vi "Demo HAL Tester LITE.vi"() -> ()   [LabVIEW 2014]
doc: "Use this template to build a producer/consumer design pattern with events to produce queue items. Use this design pattern instead of the User Interface Event Handler pattern for user interfaces when you want to execute code asynchronously in response to an event without slowing the user interface responsiveness."
uses:
  TypeDefs/HAL Config Data.ctl
  APIs/Message Queue/Enqueue Message (Single).vi
  APIs/Message Queue/Enqueue Message (Array).vi
  APIs/Message Queue/WINFAS 2 Message Queue.lvlib
  HWSyncLoop/HWSyncLoop.lvlib
  APIs/Data Queue/WINFAS 2 Data Queue.lvlib
  HWAsyncLoop/HWAsyncLoop.lvlib
panel:
  out "Asyncs":string[][](array[string])
  out "Syncs":string[](array[string])
  out "Async Data":sgl[](array[numeric])
  in  "HWAsync CMD":bool
  in  "HWSync CMD":bool
  in  "Stop Cycle":bool
  in  "Start Cycle":bool
  in  "Config":bool
  in  "LOAD DRIVER":bool
  in  "Disconnect":bool
  in  "Connect":bool
  out "UI Mssge Log":string
  out "TDX":sgl[][](graph)
  out "Encoder":sgl[](array[slide]) scale=-3600.0..3600.0
  out "DO":bool[][](array[boolean])
  out "DI":bool[][](array[boolean])
  out "TDX ALL":string[][](table)
  out "HWSyncLog 1":string
  out "HWSyncLog 2":string
  out "HWSyncLog 3":string
  out "HWSyncLog 4":string
  out "HWSyncLog 5":string
  out "HWAsyncLogAll":string
  # "Entradas Digitales (0-15)"
  # "Salidas Digitales (0-15)"
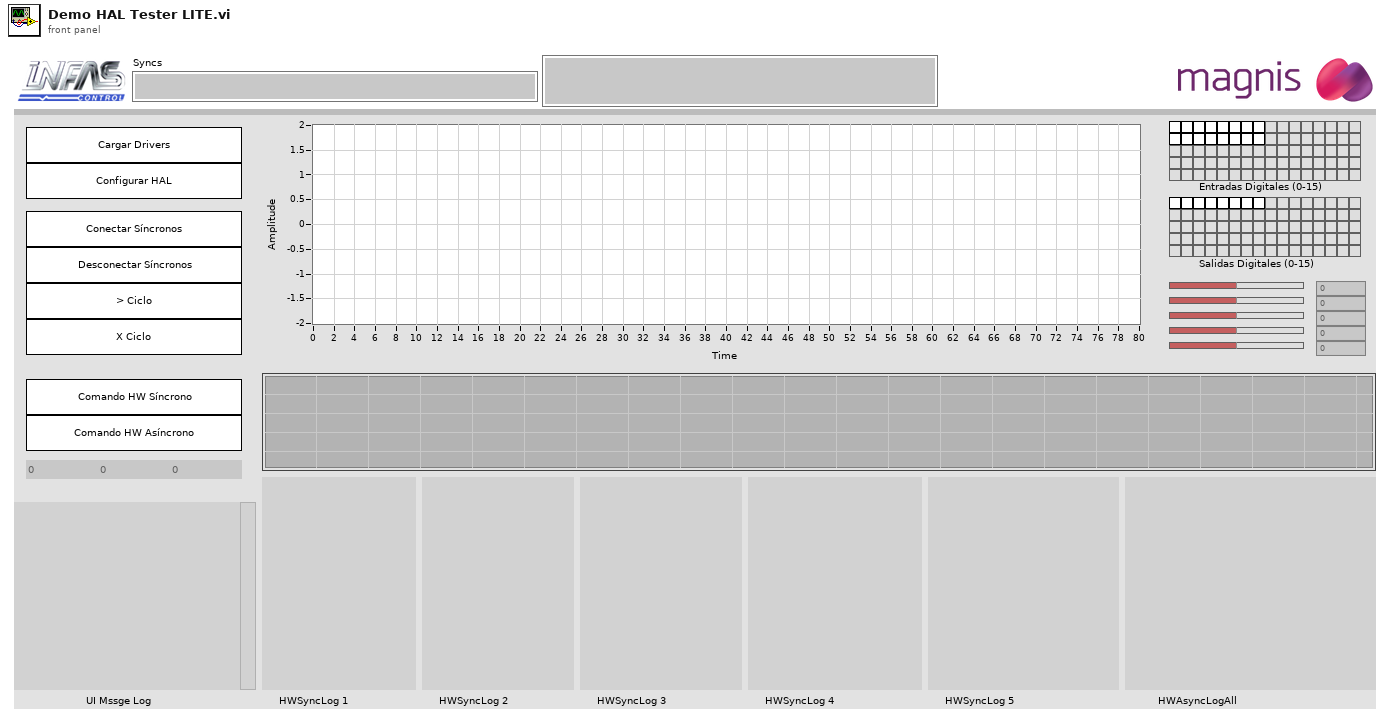
[diagram p1: front panel]
types:
  T1 = typedef "HAL Config Data.ctl" = cluster{"HWSync Index":u32, "Driver Name":string, "Channel Mask":u64}
  T2 = enum32{"invalid app kind", "Development System", "Run Time System", "Student Edition", "Embedded LabVIEW", "Evaluation", "Custom"}
  T3 = typedef "WINFAS 2 Message Queue.lvlib/All Message Queues.ctl" = cluster{"CORE":refnum<queue>, "Event UI":refnum<queue>, "Display UI":refnum<queue>, "MATH":refnum<queue>, "SEQ":refnum<queue>, "DB":refnum<queue>, "ERR":refnum<queue>, "HAL":refnum<queue>, "HWSync1":refnum<queue>, "HWSync2":refnum<queue>, "HWSync3":refnum<queue>, "HWSync4":refnum<queue>, "HWSync5":refnum<queue>, "HWAsync1":refnum<queue>, "HWAsync2":refnum<queue>, "HWAsync3":refnum<queue>, "HWAsync4":refnum<queue>, "HWAsync5":refnum<queue>, "HWAsync6":refnum<queue>, "HWAsync7":refnum<queue>, "HWAsync8":refnum<queue>, "HWAsync9":refnum<queue>, "HWAsync10":refnum<queue>}
  T4 = typedef "WINFAS 2 Data Queue.lvlib/All Data Queues Cluster.ctl" = cluster{"Queues":cluster{"ACQ HWSync1":refnum<queue>, "ACQ HWSync2":refnum<queue>, "ACQ HWSync3":refnum<queue>, "ACQ HWSync4":refnum<queue>, "ACQ HWSync5":refnum<queue>}, "Notifiers":cluster{"Control":cluster{"CTRL HWSync1":refnum<notifier>, "CTRL HWSync2":refnum<notifier>, "CTRL HWSync3":refnum<notifier>, "CTRL HWSync4":refnum<notifier>, "CTRL HWSync5":refnum<notifier>}, "Acquisition":cluster{"ACQ HWSync1":refnum<notifier>, "ACQ HWSync2":refnum<notifier>, "ACQ HWSync3":refnum<notifier>, "ACQ HWSync4":refnum<notifier>, "ACQ HWSync5":refnum<notifier>}, "Async":cluster{"ACQ HWAsync1":refnum<notifier>, "ACQ HWAsync2":refnum<notifier>, "ACQ HWAsync3":refnum<notifier>, "ACQ HWAsync4":refnum<notifier>, "ACQ HWAsync5":refnum<notifier>, "ACQ HWAsync6":refnum<notifier>, "ACQ HWAsync7":refnum<notifier>, "ACQ HWAsync8":refnum<notifier>, "ACQ HWAsync9":refnum<notifier>, "ACQ HWAsync10":refnum<notifier>}}}
  T5 = cluster{"ACQ HWSync1":refnum<notifier>, "ACQ HWSync2":refnum<notifier>, "ACQ HWSync3":refnum<notifier>, "ACQ HWSync4":refnum<notifier>, "ACQ HWSync5":refnum<notifier>}
  T6 = cluster{"CTRL HWSync1":refnum<notifier>, "CTRL HWSync2":refnum<notifier>, "CTRL HWSync3":refnum<notifier>, "CTRL HWSync4":refnum<notifier>, "CTRL HWSync5":refnum<notifier>}
  T7 = cluster{"ACQ HWSync1":refnum<queue>, "ACQ HWSync2":refnum<queue>, "ACQ HWSync3":refnum<queue>, "ACQ HWSync4":refnum<queue>, "ACQ HWSync5":refnum<queue>}
  T8 = cluster{"HWSync1":refnum<queue>, "HWSync2":refnum<queue>, "HWSync3":refnum<queue>, "HWSync4":refnum<queue>, "HWSync5":refnum<queue>}
  T9 = cluster{"HWAsync1":refnum<queue>, "HWAsync2":refnum<queue>, "HWAsync3":refnum<queue>, "HWAsync4":refnum<queue>, "HWAsync5":refnum<queue>, "HWAsync6":refnum<queue>, "HWAsync7":refnum<queue>, "HWAsync8":refnum<queue>, "HWAsync9":refnum<queue>, "HWAsync10":refnum<queue>}
  T10 = typedef "WINFAS 2 Data Queue.lvlib/Async Acquisition Data Cluster.ctl" = cluster{"Data":sgl[]}
  T11 = typedef "WINFAS 2 Data Queue.lvlib/Acquisition Data 1 Sample Cluster.ctl" = cluster{"TDX":sgl[], "Encoder":sgl}
  T12 = typedef "WINFAS 2 Data Queue.lvlib/Control Data Cluster.ctl" = cluster{"Encoder":sgl, "DI":bool[], "DO":bool[]}
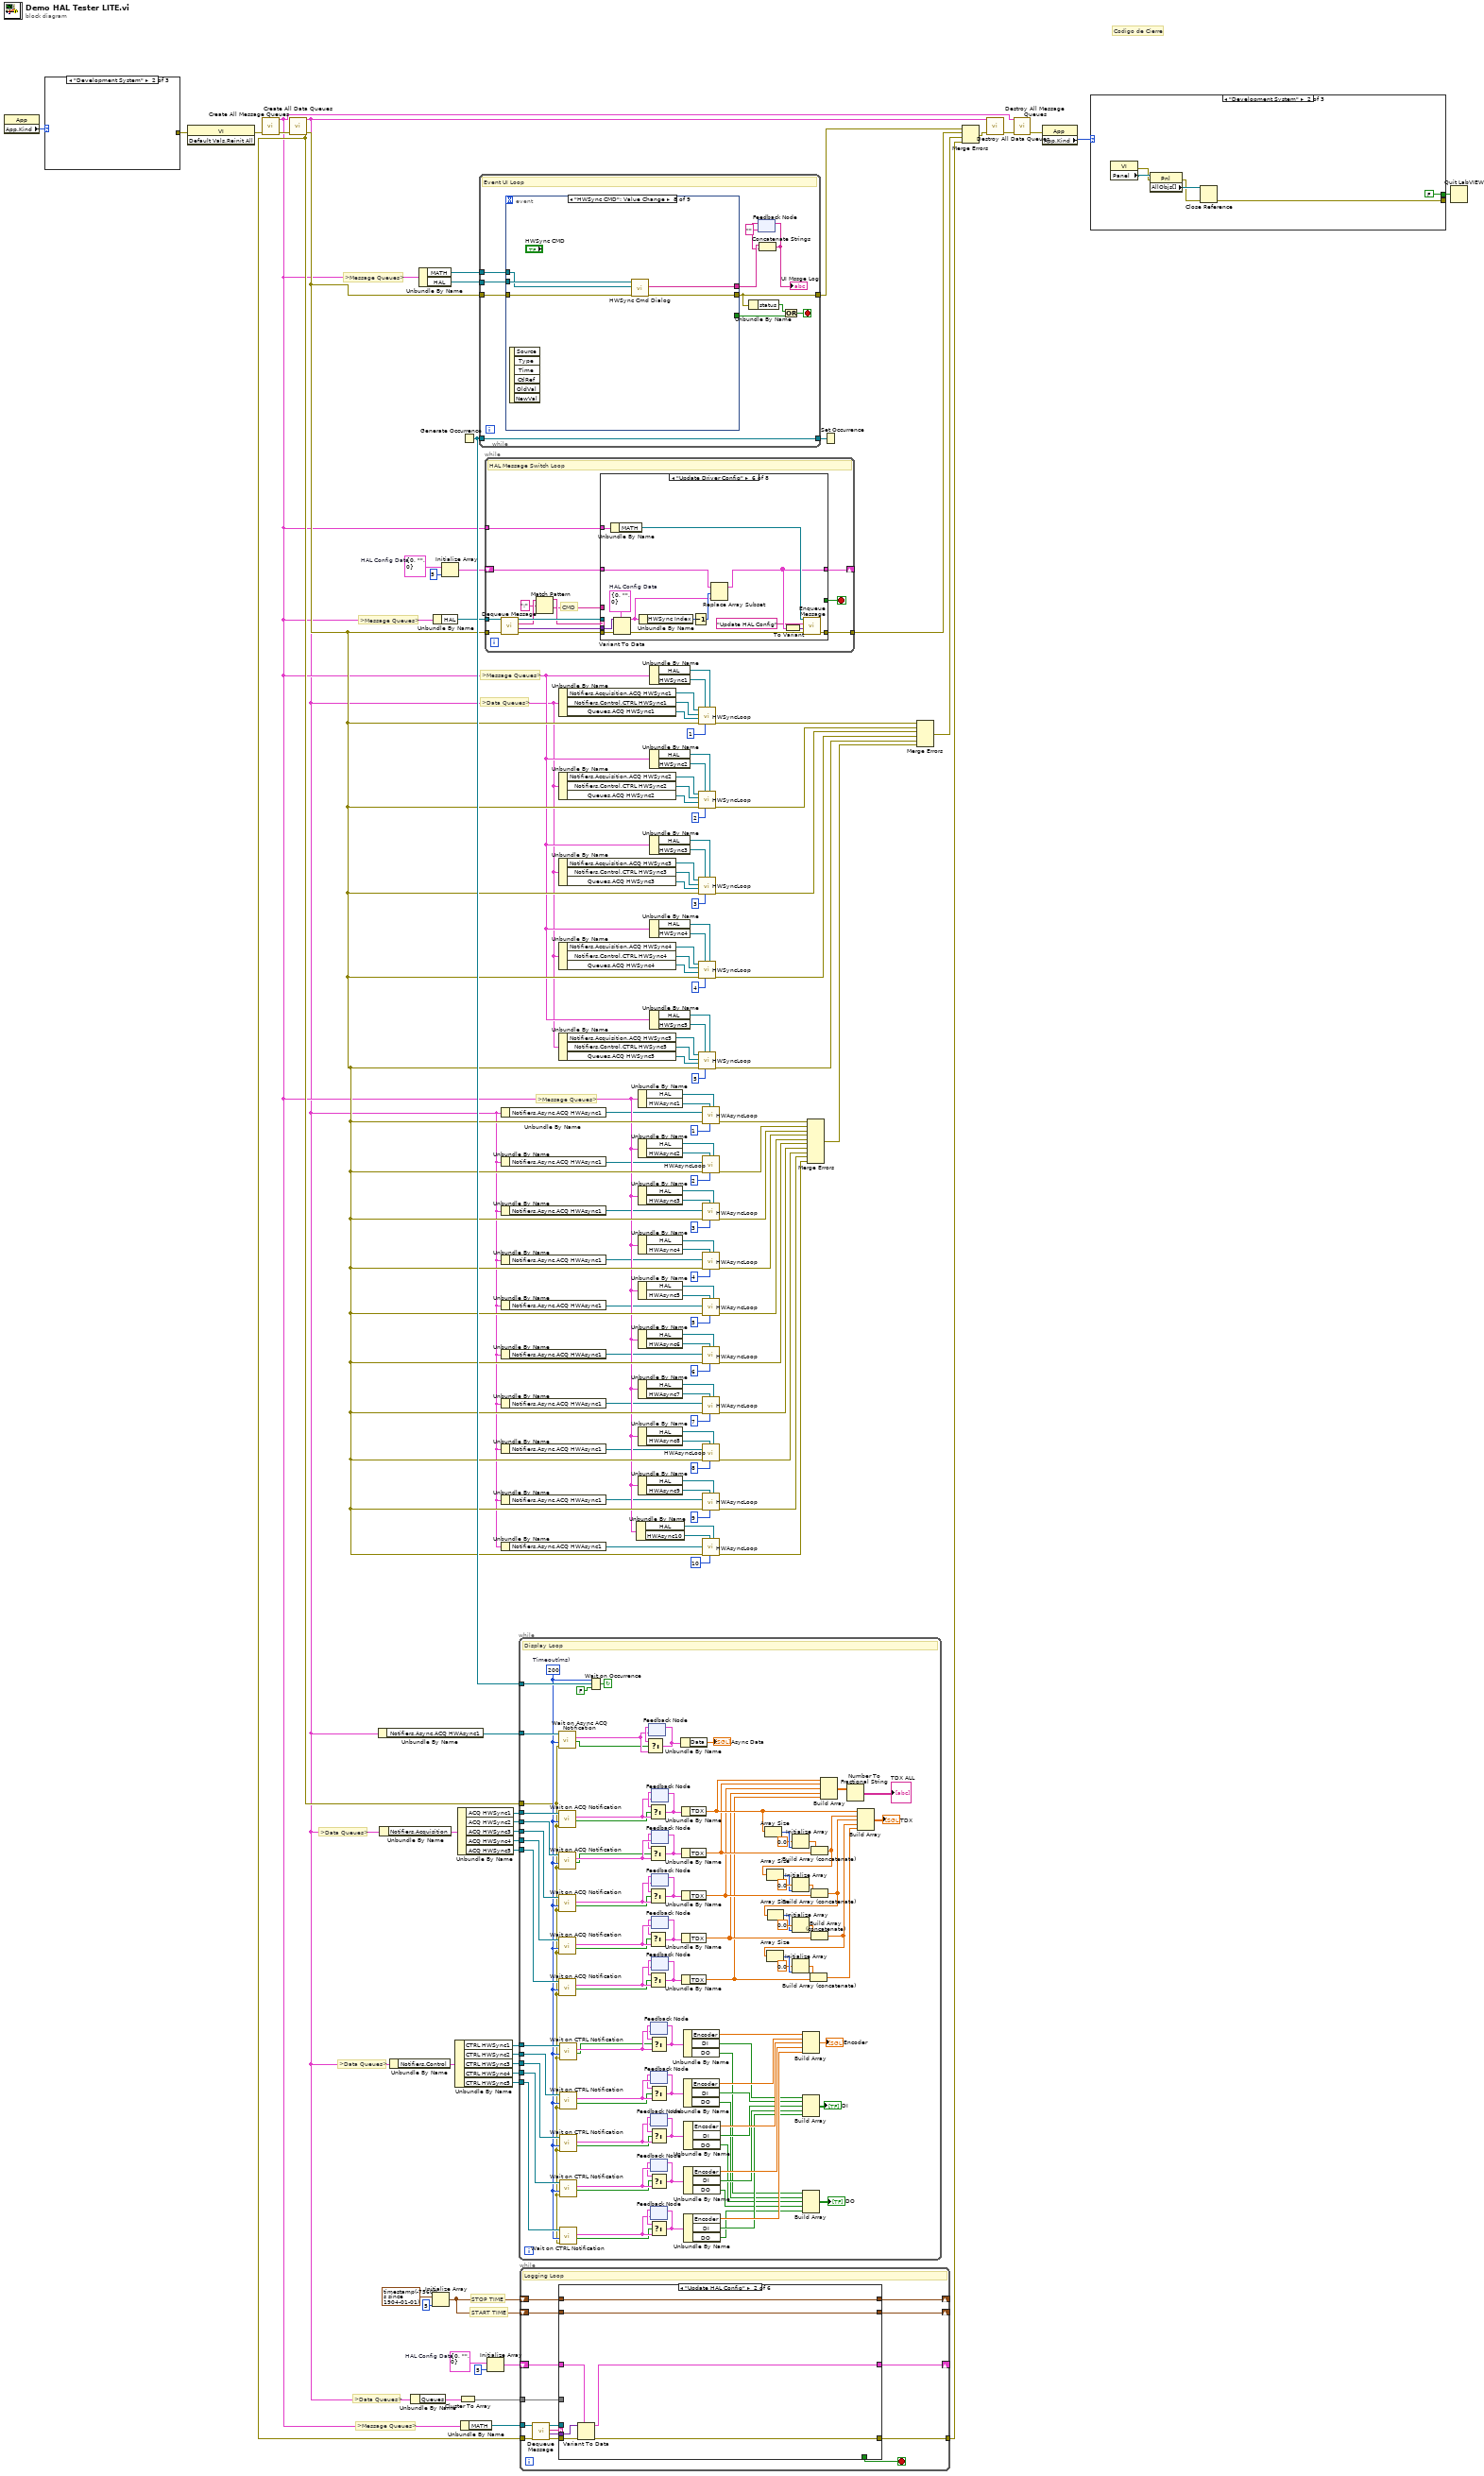
[diagram p0: block diagram]
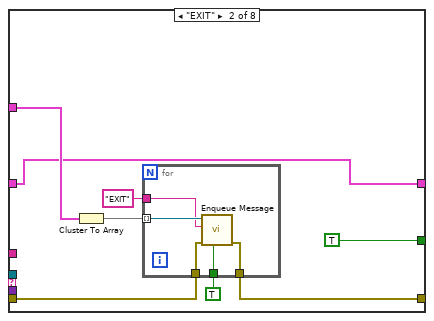
[diagram p3: hidden frame]
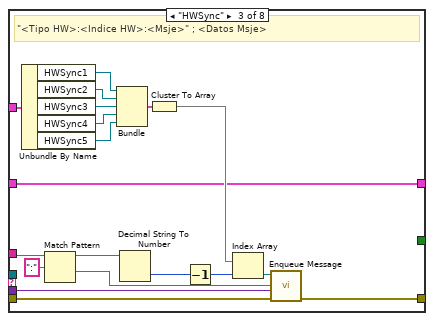
[diagram p4: hidden frame]
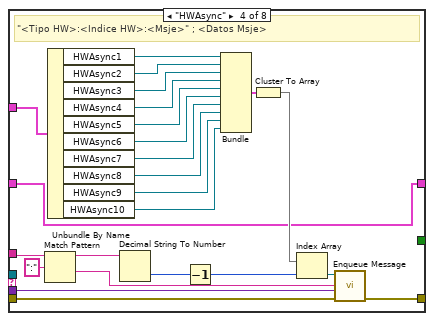
[diagram p5: hidden frame]
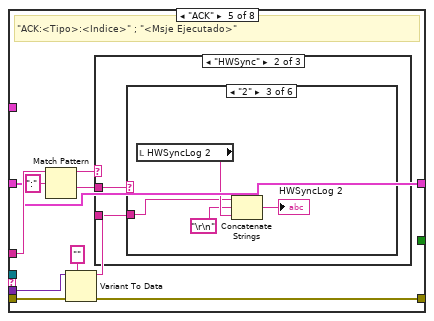
[diagram p6: hidden frame]
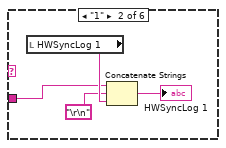
[diagram p9: hidden frame]
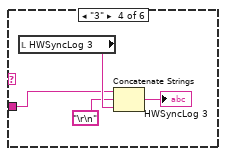
[diagram p10: hidden frame]
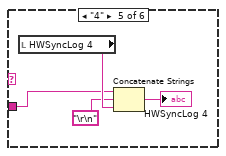
[diagram p11: hidden frame]
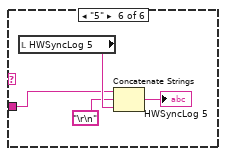
[diagram p12: hidden frame]
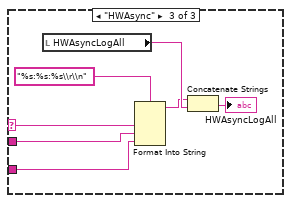
[diagram p13: hidden frame]
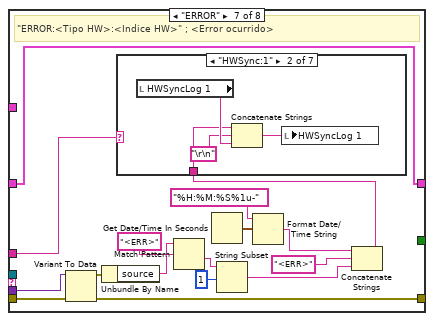
[diagram p14: hidden frame]
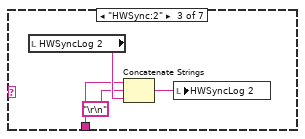
[diagram p16: hidden frame]
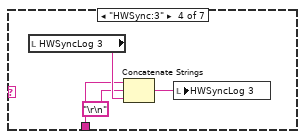
[diagram p17: hidden frame]
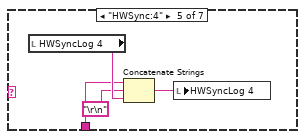
[diagram p18: hidden frame]
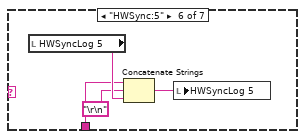
[diagram p19: hidden frame]
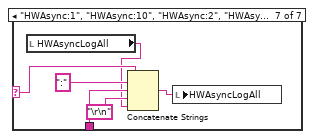
[diagram p20: hidden frame]
diagram:
  w17 = T1 {"HWSync Index"=0, "Driver Name"="", "Channel Mask"=0}  # HAL Config Data
  w20 = T1 {"HWSync Index"=0, "Driver Name"="", "Channel Mask"=0}  # HAL Config Data
  # "START TIME"
  # "STOP TIME"
  # ">Message Queues>"
  # ">Message Queues>"
  # ">Data Queues>"
  # "Codigo de Cierre"
  # ">Message Queues>"
  # ">Data Queues>"
  # ">Message Queues>"
  # ">Data Queues>"
  # ">Data Queues>"
  # ">Message Queues>"
  n1 = property class="App"() -> ("App.Kind"=w123:T2)  [unwired: 2 in, 2 out]
  n2 = case shown="\"Development System\"" w123 {
    tunnel: [_ _ w134] -> w122
    frame "invalid app kind", Default {
    }
    frame "Development System" {
    }
    frame "Run Time System" {
      w133 = FALSE ("Front Panel Window:Show Menu Bar")
      n3 = invoke class="VI" method="FP.Run-Time Position.Maximized"("Monitor"=i16 0) -> (error out=w134:errorcluster)  [unwired: 3 in, 3 out]
      n4 = property class="VI"("Front Panel.ShowMenuBar"=w133, "TB.Visible"=w133) -> ()  [unwired: 2 in, 2 out]
    }
  }
  n5 = invoke class="VI" method="Default Vals.Reinit All"(error in=w122) -> (error out=w113:errorcluster)  [unwired: 2 in, 2 out]
  n6 = call "Create All Message Queues.vi"("error in (no error)"=w113) -> ("error out"=w114:errorcluster, "Message Queues Out"=w24:T3)  [unwired: 9 in]
  n7 = call "Create All Data Queues.vi"("Error In"=w114) -> ("Error Out"=w36:errorcluster, "WINFAS 2 Data Queue.lvlib:All Data Queues Cluster"=w2:T4)  [unwired: 9 in]
  n8 = Unbundle By Name(w2) -> ("Notifiers.Async.ACQ HWAsync1"=w1:refnum<notifier>)
  n9 = Unbundle By Name(w2) -> ("Notifiers.Acquisition"=w68:T5)
  n10 = Unbundle By Name(w2) -> ("Notifiers.Control"=w67:T6)
  n11 = Unbundle By Name(w2) -> ("Queues"=w14:T7)
  n12 = Unbundle By Name(w24) -> ("MATH"=w132:refnum<queue>, "HAL"=w128:refnum<queue>)
  n13 = Initialize Array(timestamp(-75600 s since 1904-01-01) ("current time"), 5 ("dimension size")) -> (w21:timestamp[])
  n14 = Unbundle By Name(w24) -> ("HAL"=w72:refnum<queue>)
  n15 = Initialize Array(w17, 5 ("dimension size")) -> (w15:T1[])
  n16 = Unbundle By Name(w67) -> ("CTRL HWSync1"=w77:refnum<notifier>, "CTRL HWSync2"=w76:refnum<notifier>, "CTRL HWSync3"=w75:refnum<notifier>, "CTRL HWSync4"=w74:refnum<notifier>, "CTRL HWSync5"=w73:refnum<notifier>)
  n17 = Unbundle By Name(w68) -> ("ACQ HWSync1"=w118:refnum<notifier>, "ACQ HWSync2"=w81:refnum<notifier>, "ACQ HWSync3"=w80:refnum<notifier>, "ACQ HWSync4"=w79:refnum<notifier>, "ACQ HWSync5"=w78:refnum<notifier>)
  n18 = Cluster To Array(cluster=w14) -> (array=w13:refnum<queue>[])
  n19 = Unbundle By Name(w24) -> ("MATH"=w126:refnum<queue>)
  n20 = Generate Occurrence() -> (w111:refnum<k4>)
  n21 = while {
    tunnel: w132 -> [w147]
    tunnel: w128 -> [w142]
    tunnel: [w140] -> w112
    tunnel: w111 -> [w140]
    tunnel: w36 -> [w146]
    tunnel: [w144] -> w129
    stop <- w141 stop-if-true
    # "Event UI Loop"
    n22 = event shown="[7] \"HWSync CMD\": Value Change" {
      selector: _ -> [_ _ _ _ _ _ _ _ _]
      dyn-events: _ -> [_ _ _ _ _ _ _ _ _]
      timeout: _ -> [_ _ _ _ _ _ _ _ _]
      tunnel: w147 -> [w153 _ _ _ _ _ w212 w227 _]
      tunnel: w146 -> [w155 w165 w171 w180 w187 w194 w211 w231 w237]
      tunnel: [w150 w163 w170 w179 w186 w192 w216 w230 w235] -> w144
      tunnel: [TRUE ("stop") _ _ _ _ _ _ _ _] -> w145
      tunnel: w142 -> [w156 w164 w169 w178 w185 w193 w217 w229 w232]
      tunnel: [_ w162 w166 w175 w184 w189 w215 w228 w234] -> w139
      event Panel Close? {
        w154 = TRUE ("Priority Message? (F)")
        w152 = "EXIT" ("String")
        n23 = event-data() -> ()  [unwired: 1 in, 1 out]
        n24 = call-poly "Enqueue Message.vi"("Priority Message? (F)"=w154, "error in (no error)"=w155, "Message"=w152, "Message Queue"=w156) -> ("error out"=w151:errorcluster)  [unwired: 6 in, 1 out]
        n25 = call-poly "Enqueue Message.vi"("Priority Message? (F)"=w154, "error in (no error)"=w151, "Message"=w152, "Message Queue"=w153) -> ("error out"=w150:errorcluster)  [unwired: 6 in, 1 out]
        n26 = event-data("Discard?"=TRUE) -> ()  [unwired: 1 in, 1 out]
      }
      event "LOAD DRIVER": Value Change {
        n27 = event-data() -> ()  [unwired: 1 in, 1 out]
        n28 = call "Load Drivers Dialog.vi"("error in (no error)"=w165, "Message Queue in"=w164) -> ("error out"=w163:errorcluster, "Mssgs Sent"=w162:string, "Asyncs"=w160:string[], "Syncs"=→"Syncs":string[])  [unwired: 6 in]
        n29 = Reshape Array(w160, 2 ("dimension size"), 5 ("dimension size")) -> (→"Asyncs":string[][])
      }
      event "Connect": Value Change {
        w168 = string[] ["HWSync:1:Port:Open", "HWSync:2:Port:Open", "HWSync:3:Port:Open", "HWSync:4:Port:Open", "HWSync:5:Port:Open"] ("Message Array")
        n30 = event-data() -> ()  [unwired: 1 in, 1 out]
        n31 = for {
          tunnel: [w174] -> w167 mode=indexing
          tunnel: w168 -> [w173] mode=indexing
          n32 = Concatenate Strings(w173, "\r\n") -> (w174:string)
        }
        n33 = call-poly "Enqueue Message.vi"("error in (no error)"=w171, "Message Array"=w168, "Message Queue"=w169) -> ("error out"=w170:errorcluster)  [unwired: 7 in, 1 out]
        n34 = Concatenate Strings(w167) -> (w166:string)
      }
      event "Disconnect": Value Change {
        w176 = string[] ["HWSync:1:Port:Close", "HWSync:2:Port:Close", "HWSync:3:Port:Close", "HWSync:4:Port:Close", "HWSync:5:Port:Close"] ("Message Array")
        n35 = event-data() -> ()  [unwired: 1 in, 1 out]
        n36 = for {
          tunnel: [w183] -> w177 mode=indexing
          tunnel: w176 -> [w182] mode=indexing
          n37 = Concatenate Strings(w182, "\r\n") -> (w183:string)
        }
        n38 = call-poly "Enqueue Message.vi"("error in (no error)"=w180, "Message Array"=w176, "Message Queue"=w178) -> ("error out"=w179:errorcluster)  [unwired: 7 in, 1 out]
        n39 = Concatenate Strings(w177) -> (w175:string)
      }
      event "Config": Value Change {
        n40 = event-data() -> ()  [unwired: 1 in, 1 out]
        n41 = call "Config Select Dialog.vi"("Error In"=w187, "Message Queue"=w185) -> ("Error Out"=w186:errorcluster, "Msg out"=w184:string)  [unwired: 8 in]
      }
      event "Start Cycle": Value Change {
        n42 = event-data() -> ()  [unwired: 1 in, 2 out]
        n43 = for {
          N: 5 -> [_]
          tunnel: w193 -> [w208]
          shift-right: [w207] -> w192
          shift-left: w194 -> [w209]
          tunnel: [w198] -> w190 mode=concatenating
          i -> [w206]
          n44 = Increment(x=w206) -> (x+1=w202:i32)
          n45 = Format Into String(format string="HWSync:%d:Auto-Refresh:Init" ("String"), w202) -> (resulting string=w201:string)  [unwired: 2 in, 1 out]
          n46 = Format Into String(format string="HWSync:%d:Auto-Refresh:Start" ("String"), w202) -> (resulting string=w200:string)  [unwired: 2 in, 1 out]
          n47 = Format Into String(format string="HWSync:%d:Diagnostic:Cycle" ("String"), w202) -> (resulting string=w199:string)  [unwired: 2 in, 1 out]
          n48 = Build Array(w201, w200, w199) -> (w198:string[])
          n49 = call-poly "Enqueue Message.vi"("error in (no error)"=w209, "Message Array"=w198, "Message Queue"=w208) -> ("error out"=w207:errorcluster)  [unwired: 7 in, 1 out]
        }
        n50 = for {
          tunnel: [w197] -> w191 mode=indexing
          tunnel: w190 -> [w196] mode=indexing
          n51 = Concatenate Strings(w196, "\r\n") -> (w197:string)
        }
        n52 = Concatenate Strings(w191) -> (w189:string)
      }
      event "Stop Cycle": Value Change {
        n53 = event-data() -> ()  [unwired: 1 in, 1 out]
        n54 = for {
          N: 5 -> [_]
          tunnel: w217 -> [w225]
          shift-right: [w224] -> w216
          shift-left: w211 -> [w226]
          tunnel: [w218] -> w214 mode=indexing
          i -> [w223]
          n55 = Increment(x=w223) -> (x+1=w221:i32)
          n56 = Format Into String(format string="HWSync:%d:Auto-Refresh:Stop" ("String"), w221) -> (resulting string=w219:string)  [unwired: 2 in, 1 out]
          n57 = call-poly "Enqueue Message.vi"("error in (no error)"=w226, "Message"=w219, "Message Queue"=w225) -> ("error out"=w224:errorcluster)  [unwired: 7 in, 1 out]
          n58 = Concatenate Strings(w219, "\r\n") -> (w218:string)
        }
        n59 = call-poly "Enqueue Message.vi"("error in (no error)"=w211, "Message"="Open Log File", "Message Queue"=w212) -> ()  [unwired: 7 in, 2 out]
        n60 = Concatenate Strings(w214) -> (w215:string)
      }
      event "HWSync CMD": Value Change {
        n61 = event-data() -> ()  [unwired: 1 in, 6 out]
        n62 = call "HWSync Cmd Dialog.vi"("error in (no error)"=w231, "Log Queue"=w227, "Hal Queue in"=w229) -> ("error out"=w230:errorcluster, "Msg out"=w228:string)  [unwired: 7 in]
      }
      event "HWAsync CMD": Value Change {
        n63 = event-data() -> ()  [unwired: 1 in, 6 out]
        n64 = call "HWAsync Cmd Dialog.vi"("error in (no error)"=w237) -> ("error out"=w236:errorcluster, "Msg out"=w233:string)  [unwired: 9 in]
        n65 = call "HWAsync Cmd END Dialog.vi"("error in (no error)"=w236, "Msg in"=w233, "Message Queue"=w232) -> ("error out"=w235:errorcluster, "Msg out"=w234:string)  [unwired: 7 in]
      }
    }
    n66 = Unbundle By Name(w144) -> ("status"=w143:bool)
    n67 = feedback #1("") -> (w138:string)
    n68 = Concatenate Strings(w139, w138) -> (w137:string)
    "UI Mssge Log" <- w137
    n69 = feedback-in #1(w137) -> ()
    n70 = Or(x=w143, y=w145) -> (x .or. y?=w141:bool)
  }
  n71 = while {
    tunnel: w72 -> [w251]
    tunnel: w36 -> [w250]
    tunnel: [w242] -> w69
    tunnel: w24 -> [w241]
    shift-right: [w238] -> _
    shift-left: w15 -> [w239]
    stop <- w246 stop-if-true
    # "CMD"
    # "HAL Message Switch Loop"
    n72 = call "Dequeue Message.vi"("error in (no error)"=w250, "Message Queue"=w251) -> ("error out"=w249:errorcluster, "Message Data"=w248:variant, "Message"=w245:string, "dup Message Queue"=w247:refnum<queue>)  [unwired: 6 in]
    n73 = Match Pattern(string=w245, regular expression=":") -> (before substring=w243:string, after substring=w240:string)  [unwired: 1 in, 2 out]
    n74 = case shown="\"Update Driver Config\"" w243 {
      tunnel: w249 -> [w253 w260 w285 w309 w319 w362 w369 w416]
      tunnel: w248 -> [_ _ w283 w307 w318 w361 w378 w421]
      tunnel: w247 -> [_ _ _ _ _ _ _ _]
      tunnel: [_ TRUE _ _ _ _ _ _] -> w246
      tunnel: [w253 w259 w284 w308 w317 w354 w377 w420] -> w242
      tunnel: w241 -> [_ w257 w282 w306 _ w353 _ _]
      tunnel: w240 -> [_ _ w275 w300 w313 _ w366 w414]
      tunnel: w239 -> [w252 w254 w267 w286 w310 w356 w365 w413]
      tunnel: [w252 w254 w267 w286 w310 w350 w365 w413] -> w238
      frame Default {
      }
      frame "EXIT" {
        n75 = Cluster To Array(cluster=w257) -> (array=w256:refnum<queue>[])
        n76 = for {
          tunnel: w256 -> [w264] mode=indexing
          tunnel: "EXIT" ("regular expression") -> [w263]
          tunnel: w260 -> [w266]
          tunnel: [w265] -> w259
          tunnel: TRUE -> [w262]
          n77 = call-poly "Enqueue Message.vi"("Priority Message? (F)"=w262, "error in (no error)"=w266, "Message"=w263, "Message Queue"=w264) -> ("error out"=w265:errorcluster)  [unwired: 6 in, 1 out]
        }
      }
      frame "HWSync" {
        # "\"<Tipo HW>:<Indice HW>:<Msje>\" ; <Datos Msje>"
        n78 = Unbundle By Name(w282) -> ("HWSync1"=w278:refnum<queue>, "HWSync2"=w280:refnum<queue>, "HWSync3"=w281:refnum<queue>, "HWSync4"=w279:refnum<queue>, "HWSync5"=w277:refnum<queue>)
        n79 = Match Pattern(string=w275, regular expression=":") -> (before substring=w272:string, after substring=w270:string)  [unwired: 1 in, 2 out]
        n80 = Bundle("HWSync1"=w278, "HWSync2"=w280, "HWSync3"=w281, "HWSync4"=w279, "HWSync5"=w277) -> (w274:T8)  [unwired: 1 in]
        n81 = Decimal String To Number(string=w272) -> (number=w268:i32)  [unwired: 2 in, 1 out]
        n82 = Cluster To Array(cluster=w274) -> (array=w273:refnum<queue>[])
        n83 = Decrement(x=w268) -> (x-1=w269:i32)
        n84 = Index Array(array=w273, index=w269) -> (element=w271:refnum<queue>)
        n85 = call-poly "Enqueue Message.vi"("error in (no error)"=w285, "Message Data"=w283, "Message"=w270, "Message Queue"=w271) -> ("error out"=w284:errorcluster)  [unwired: 6 in, 1 out]
      }
      frame "HWAsync" {
        # "\"<Tipo HW>:<Indice HW>:<Msje>\" ; <Datos Msje>"
        n86 = Match Pattern(string=w300, regular expression=":") -> (before substring=w297:string, after substring=w295:string)  [unwired: 1 in, 2 out]
        n87 = Unbundle By Name(w306) -> ("HWAsync1"=w303:refnum<queue>, "HWAsync2"=w287:refnum<queue>, "HWAsync3"=w305:refnum<queue>, "HWAsync4"=w304:refnum<queue>, "HWAsync5"=w302:refnum<queue>, "HWAsync6"=w288:refnum<queue>, "HWAsync7"=w289:refnum<queue>, "HWAsync8"=w290:refnum<queue>, "HWAsync9"=w291:refnum<queue>, "HWAsync10"=w292:refnum<queue>)
        n88 = Decimal String To Number(string=w297) -> (number=w293:i32)  [unwired: 2 in, 1 out]
        n89 = Decrement(x=w293) -> (x-1=w294:i32)
        n90 = Bundle("HWAsync1"=w303, "HWAsync2"=w287, "HWAsync3"=w305, "HWAsync4"=w304, "HWAsync5"=w302, "HWAsync6"=w288, "HWAsync7"=w289, "HWAsync8"=w290, "HWAsync9"=w291, "HWAsync10"=w292) -> (w299:T9)  [unwired: 1 in]
        n91 = Cluster To Array(cluster=w299) -> (array=w298:refnum<queue>[])
        n92 = Index Array(array=w298, index=w294) -> (element=w296:refnum<queue>)
        n93 = call-poly "Enqueue Message.vi"("error in (no error)"=w309, "Message Data"=w307, "Message"=w295, "Message Queue"=w296) -> ("error out"=w308:errorcluster)  [unwired: 6 in, 1 out]
      }
      frame "ACK" {
        # "\"ACK:<Tipo>:<Indice>\" ; \"<Msje Ejecutado>\""
        n94 = Match Pattern(string=w313, regular expression=":") -> (before substring=w314:string, after substring=w311:string)  [unwired: 1 in, 2 out]
        n95 = Variant To Data(error in=w319, type="", Variant=w318) -> (data=w316:string, error out=w317:errorcluster)
        n96 = case shown="\"HWSync\"" w314 {
          selector: w314 -> [_ _ w347]
          tunnel: w316 -> [_ w321 w345]
          tunnel: w311 -> [_ w320 w346]
          frame Default {
          }
          frame "HWSync" {
            n97 = case shown="\"2\"" w320 {
              tunnel: w321 -> [_ w322 w328 w332 w336 w340]
              frame Default {
              }
              frame "1" {
                n98 = local read "HWSyncLog 1"() -> (w325:string)
                n99 = Concatenate Strings(w322, "\r\n", w325) -> (→"HWSyncLog 1":string)
              }
              frame "2" {
                n100 = local read "HWSyncLog 2"() -> (w329:string)
                n101 = Concatenate Strings(w328, "\r\n", w329) -> (→"HWSyncLog 2":string)
              }
              frame "3" {
                n102 = local read "HWSyncLog 3"() -> (w333:string)
                n103 = Concatenate Strings(w332, "\r\n", w333) -> (→"HWSyncLog 3":string)
              }
              frame "4" {
                n104 = local read "HWSyncLog 4"() -> (w337:string)
                n105 = Concatenate Strings(w336, "\r\n", w337) -> (→"HWSyncLog 4":string)
              }
              frame "5" {
                n106 = local read "HWSyncLog 5"() -> (w341:string)
                n107 = Concatenate Strings(w340, "\r\n", w341) -> (→"HWSyncLog 5":string)
              }
            }
          }
          frame "HWAsync" {
            n108 = local read "HWAsyncLogAll"() -> (w344:string)
            n109 = Format Into String(format string="%s:%s:%s\\r\\n", w347, w346, w345) -> (resulting string=w343:string)  [unwired: 2 in, 1 out]
            n110 = Concatenate Strings(w343, w344) -> (→"HWAsyncLogAll":string)
          }
        }
      }
      frame "Update Driver Config" {
        w360 = T1 {"HWSync Index"=0, "Driver Name"="", "Channel Mask"=0}  # HAL Config Data
        n111 = Unbundle By Name(w353) -> ("MATH"=w352:refnum<queue>)
        n112 = Variant To Data(error in=w362, type=w360, Variant=w361) -> (data=w357:T1, error out=w355:errorcluster)
        n113 = Unbundle By Name(w357) -> ("HWSync Index"=w359:u32)
        n114 = Decrement(x=w359) -> (x-1=w358:u32)
        n115 = Replace Array Subset(array=w356, new element=w357, index=w358) -> (w350:T1[])
        n116 = To Variant(anything=w350) -> (Variant=w351:variant)
        n117 = call-poly "Enqueue Message.vi"("error in (no error)"=w355, "Message Data"=w351, "Message"="Update HAL Config" ("regular expression"), "Message Queue"=w352) -> ("error out"=w354:errorcluster)  [unwired: 6 in, 1 out]
      }
      frame "ERROR" {
        # "\"ERROR:<Tipo HW>:<Indice HW>\" ; <Error ocurrido>"
        n118 = Variant To Data(error in=w369, type=w369, Variant=w378) -> (data=w368:errorcluster, error out=w377:errorcluster)
        n119 = Unbundle By Name(w368) -> ("source"=w375:string)
        n120 = Match Pattern(string=w375, regular expression="<ERR>") -> (after substring=w371:string)  [unwired: 1 in, 3 out]
        n121 = Get Date/Time In Seconds() -> (seconds since 1Jan1904=w374:timestamp)
        n122 = String Subset(string=w371, offset (0)=1) -> (substring=w364:string)  [unwired: 1 in]
        n123 = Format Date/Time String(time format string (%c)="%H:%M:%S%1u-", seconds (now)=w374) -> (date/time string=w372:string)  [unwired: 1 in]
        n124 = Concatenate Strings(w372, "<ERR>" ("string"), w364) -> (w367:string)
        n125 = case shown="\"HWSync:1\"" w366 {
          selector: w366 -> [_ _ _ _ _ _ w402]
          tunnel: w367 -> [_ w381 w385 w389 w393 w397 w404]
          frame Default {
          }
          frame "HWSync:1" {
            n126 = local read "HWSyncLog 1"() -> (w382:string)
            n127 = Concatenate Strings(w381, "\r\n", w382) -> (w379:string)
            n128 = local write "HWSyncLog 1"(w379) -> ()
          }
          frame "HWSync:2" {
            n129 = local read "HWSyncLog 2"() -> (w386:string)
            n130 = Concatenate Strings(w385, "\r\n", w386) -> (w383:string)
            n131 = local write "HWSyncLog 2"(w383) -> ()
          }
          frame "HWSync:3" {
            n132 = local read "HWSyncLog 3"() -> (w390:string)
            n133 = Concatenate Strings(w389, "\r\n", w390) -> (w387:string)
            n134 = local write "HWSyncLog 3"(w387) -> ()
          }
          frame "HWSync:4" {
            n135 = local read "HWSyncLog 4"() -> (w394:string)
            n136 = Concatenate Strings(w393, "\r\n", w394) -> (w391:string)
            n137 = local write "HWSyncLog 4"(w391) -> ()
          }
          frame "HWSync:5" {
            n138 = local read "HWSyncLog 5"() -> (w398:string)
            n139 = Concatenate Strings(w397, "\r\n", w398) -> (w395:string)
            n140 = local write "HWSyncLog 5"(w395) -> ()
          }
          frame "HWAsync:1", "HWAsync:10", "HWAsync:2", "HWAsync:3", "HWAsync:4", "HWAsync:5", "HWAsync:6", "HWAsync:7", "HWAsync:8", "HWAsync:9" {
            n141 = local read "HWAsyncLogAll"() -> (w399:string)
            n142 = Concatenate Strings(w402, ":" ("string"), w404, "\r\n", w399) -> (w400:string)
            n143 = local write "HWAsyncLogAll"(w400) -> ()
          }
        }
      }
      frame "WARNING" {
        # "\"WARNING:<Tipo HW>:<Indice HW>\" ; <Advertencia ocurrida>"
        n144 = Variant To Data(error in=w416, type=w416, Variant=w421) -> (data=w411:errorcluster, error out=w420:errorcluster)
        n145 = Unbundle By Name(w411) -> ("code"=w406:i32, "source"=w410:string)
        n146 = Match Pattern(string=w410, regular expression="<ERR>") -> (after substring=w408:string)  [unwired: 1 in, 3 out]
        n147 = Pick Line(multi-line string=w408, line index=2) -> (output string=w407:string)  [unwired: 1 in]
        n148 = Get Date/Time In Seconds() -> (seconds since 1Jan1904=w419:timestamp)
        n149 = Format Date/Time String(time format string (%c)="%H:%M:%S%1u-", seconds (now)=w419) -> (date/time string=w417:string)  [unwired: 1 in]
        n150 = Number To Decimal String(number=w406) -> (decimal integer string=w412:string)  [unwired: 1 in]
        n151 = Concatenate Strings(w417, w407, w412) -> (w415:string)
        n152 = case shown="\"HWSync:1\"" w414 {
          selector: w414 -> [_ _ _ _ _ _ w445]
          tunnel: w415 -> [_ w424 w428 w432 w436 w440 w447]
          frame Default {
          }
          frame "HWSync:1" {
            n153 = local read "HWSyncLog 1"() -> (w425:string)
            n154 = Concatenate Strings(w424, "\r\n", w425) -> (w422:string)
            n155 = local write "HWSyncLog 1"(w422) -> ()
          }
          frame "HWSync:2" {
            n156 = local read "HWSyncLog 2"() -> (w429:string)
            n157 = Concatenate Strings(w428, "\r\n", w429) -> (w426:string)
            n158 = local write "HWSyncLog 2"(w426) -> ()
          }
          frame "HWSync:3" {
            n159 = local read "HWSyncLog 3"() -> (w433:string)
            n160 = Concatenate Strings(w432, "\r\n", w433) -> (w430:string)
            n161 = local write "HWSyncLog 3"(w430) -> ()
          }
          frame "HWSync:4" {
            n162 = local read "HWSyncLog 4"() -> (w437:string)
            n163 = Concatenate Strings(w436, "\r\n", w437) -> (w434:string)
            n164 = local write "HWSyncLog 4"(w434) -> ()
          }
          frame "HWSync:5" {
            n165 = local read "HWSyncLog 5"() -> (w441:string)
            n166 = Concatenate Strings(w440, "\r\n", w441) -> (w438:string)
            n167 = local write "HWSyncLog 5"(w438) -> ()
          }
          frame "HWAsync:1", "HWAsync:10", "HWAsync:2", "HWAsync:3", "HWAsync:4", "HWAsync:5", "HWAsync:6", "HWAsync:7", "HWAsync:8", "HWAsync:9" {
            n168 = local read "HWAsyncLogAll"() -> (w442:string)
            n169 = Concatenate Strings(w445, ":" ("string"), w447, "\r\n", w442) -> (w443:string)
            n170 = local write "HWAsyncLogAll"(w443) -> ()
          }
        }
      }
    }
  }
  n171 = Initialize Array(w20, 5 ("dimension size")) -> (w18:T1[])
  n172 = Unbundle By Name(w2) -> ("Notifiers.Async.ACQ HWAsync1"=w12:refnum<notifier>)
  n173 = Unbundle By Name(w2) -> ("Notifiers.Async.ACQ HWAsync1"=w11:refnum<notifier>)
  n174 = Unbundle By Name(w2) -> ("Notifiers.Async.ACQ HWAsync1"=w10:refnum<notifier>)
  n175 = Unbundle By Name(w2) -> ("Notifiers.Async.ACQ HWAsync1"=w9:refnum<notifier>)
  n176 = Unbundle By Name(w2) -> ("Notifiers.Async.ACQ HWAsync1"=w8:refnum<notifier>)
  n177 = Unbundle By Name(w2) -> ("Notifiers.Async.ACQ HWAsync1"=w7:refnum<notifier>)
  n178 = Unbundle By Name(w2) -> ("Notifiers.Async.ACQ HWAsync1"=w6:refnum<notifier>)
  n179 = Unbundle By Name(w2) -> ("Notifiers.Async.ACQ HWAsync1"=w5:refnum<notifier>)
  n180 = Unbundle By Name(w2) -> ("Notifiers.Async.ACQ HWAsync1"=w4:refnum<notifier>)
  n181 = Unbundle By Name(w2) -> ("Notifiers.Async.ACQ HWAsync1"=w3:refnum<notifier>)
  n182 = while {
    tunnel: w118 -> [w550]
    tunnel: w111 -> [w544]
    tunnel: w81 -> [w529]
    tunnel: w80 -> [w528]
    tunnel: w79 -> [w527]
    tunnel: w78 -> [w526]
    tunnel: w36 -> [w463]
    tunnel: w77 -> [w495]
    tunnel: w76 -> [w494]
    tunnel: w75 -> [w493]
    tunnel: w74 -> [w492]
    tunnel: w73 -> [w491]
    tunnel: w1 -> [w465]
    stop <- w545 continue-if-true
    w464 = 200  # Timeout(ms)
    # "Display Loop"
    n183 = call "Wait on Async ACQ Notification.vi"("error in (no error)"=w463, "timeout in ms (-1)"=w464, "Async ACQ Notifier in"=w465) -> ("timed out?"=w458:bool, "Async ACQ"=w461:T10)  [unwired: 5 in, 2 out]
    n184 = call "Wait on ACQ Notification.vi"("error in (no error)"=w463, "timeout in ms (-1)"=w464, "ACQ Data Notifier in"=w550) -> ("timed out?"=w457:bool, "1 Sample"=w543:T11)  [unwired: 5 in, 2 out]
    n185 = call "Wait on ACQ Notification.vi"("error in (no error)"=w463, "timeout in ms (-1)"=w464, "ACQ Data Notifier in"=w529) -> ("timed out?"=w456:bool, "1 Sample"=w541:T11)  [unwired: 5 in, 2 out]
    n186 = call "Wait on ACQ Notification.vi"("error in (no error)"=w463, "timeout in ms (-1)"=w464, "ACQ Data Notifier in"=w528) -> ("timed out?"=w455:bool, "1 Sample"=w536:T11)  [unwired: 5 in, 2 out]
    n187 = call "Wait on ACQ Notification.vi"("error in (no error)"=w463, "timeout in ms (-1)"=w464, "ACQ Data Notifier in"=w527) -> ("timed out?"=w454:bool, "1 Sample"=w535:T11)  [unwired: 5 in, 2 out]
    n188 = call "Wait on ACQ Notification.vi"("error in (no error)"=w463, "timeout in ms (-1)"=w464, "ACQ Data Notifier in"=w526) -> ("timed out?"=w453:bool, "1 Sample"=w530:T11)  [unwired: 5 in, 2 out]
    n189 = call "Wait on CTRL Notification.vi"("error in (no error)"=w463, "timeout in ms (-1)"=w464, "CTRL Data Notifier in"=w495) -> ("timed out?"=w452:bool, "Control Data"=w542:T12)  [unwired: 5 in, 2 out]
    n190 = call "Wait on CTRL Notification.vi"("error in (no error)"=w463, "timeout in ms (-1)"=w464, "CTRL Data Notifier in"=w494) -> ("timed out?"=w451:bool, "Control Data"=w523:T12)  [unwired: 5 in, 2 out]
    n191 = call "Wait on CTRL Notification.vi"("error in (no error)"=w463, "timeout in ms (-1)"=w464, "CTRL Data Notifier in"=w493) -> ("timed out?"=w450:bool, "Control Data"=w518:T12)  [unwired: 5 in, 2 out]
    n192 = call "Wait on CTRL Notification.vi"("error in (no error)"=w463, "timeout in ms (-1)"=w464, "CTRL Data Notifier in"=w492) -> ("timed out?"=w449:bool, "Control Data"=w517:T12)  [unwired: 5 in, 2 out]
    n193 = call "Wait on CTRL Notification.vi"("error in (no error)"=w463, "timeout in ms (-1)"=w464, "CTRL Data Notifier in"=w491) -> ("timed out?"=w448:bool, "Control Data"=w512:T12)  [unwired: 5 in, 2 out]
    n194 = Wait on Occurrence(1:FALSE ("ignore previous (T)"), 2:w544, 3:w464) -> (0:w545:bool)
    n195 = feedback #2(w461) -> (w462:T10)
    n196 = Select(t=w462, s=w458, f=w461) -> (s? t:f=w460:T10)
    n197 = feedback-in #2(w460) -> ()
    n198 = feedback #3(w542) -> (w549:T12)
    n199 = Select(t=w549, s=w452, f=w542) -> (s? t:f=w548:T12)
    n200 = feedback-in #3(w548) -> ()
    n201 = feedback #4(w523) -> (w521:T12)
    n202 = Select(t=w521, s=w451, f=w523) -> (s? t:f=w522:T12)
    n203 = feedback-in #4(w522) -> ()
    n204 = feedback #5(w518) -> (w520:T12)
    n205 = Select(t=w520, s=w450, f=w518) -> (s? t:f=w519:T12)
    n206 = feedback-in #5(w519) -> ()
    n207 = feedback #6(w517) -> (w515:T12)
    n208 = Select(t=w515, s=w449, f=w517) -> (s? t:f=w516:T12)
    n209 = feedback-in #6(w516) -> ()
    n210 = feedback #7(w512) -> (w514:T12)
    n211 = Select(t=w514, s=w448, f=w512) -> (s? t:f=w513:T12)
    n212 = feedback-in #7(w513) -> ()
    n213 = feedback #8(w543) -> (w547:T11)
    n214 = Select(t=w547, s=w457, f=w543) -> (s? t:f=w546:T11)
    n215 = feedback-in #8(w546) -> ()
    n216 = feedback #9(w541) -> (w539:T11)
    n217 = Select(t=w539, s=w456, f=w541) -> (s? t:f=w540:T11)
    n218 = feedback-in #9(w540) -> ()
    n219 = feedback #10(w536) -> (w538:T11)
    n220 = Select(t=w538, s=w455, f=w536) -> (s? t:f=w537:T11)
    n221 = feedback-in #10(w537) -> ()
    n222 = feedback #11(w535) -> (w533:T11)
    n223 = Select(t=w533, s=w454, f=w535) -> (s? t:f=w534:T11)
    n224 = feedback-in #11(w534) -> ()
    n225 = feedback #12(w530) -> (w532:T11)
    n226 = Select(t=w532, s=w453, f=w530) -> (s? t:f=w531:T11)
    n227 = feedback-in #12(w531) -> ()
    n228 = Unbundle By Name(w460) -> ("Data"=→"Async Data":sgl[])
    n229 = Unbundle By Name(w546) -> ("TDX"=w473:sgl[])
    n230 = Unbundle By Name(w540) -> ("TDX"=w472:sgl[])
    n231 = Unbundle By Name(w537) -> ("TDX"=w471:sgl[])
    n232 = Unbundle By Name(w534) -> ("TDX"=w470:sgl[])
    n233 = Unbundle By Name(w531) -> ("TDX"=w469:sgl[])
    n234 = Unbundle By Name(w548) -> ("Encoder"=w525:sgl, "DI"=w507:bool[], "DO"=w499:bool[])
    n235 = Unbundle By Name(w522) -> ("Encoder"=w511:sgl, "DI"=w506:bool[], "DO"=w500:bool[])
    n236 = Unbundle By Name(w519) -> ("Encoder"=w510:sgl, "DI"=w505:bool[], "DO"=w501:bool[])
    n237 = Unbundle By Name(w516) -> ("Encoder"=w509:sgl, "DI"=w504:bool[], "DO"=w498:bool[])
    n238 = Unbundle By Name(w513) -> ("Encoder"=w508:sgl, "DI"=w503:bool[], "DO"=w497:bool[])
    n239 = Array Size(array=w473) -> (size(s)=w488:i32)
    n240 = Initialize Array(sgl 0.0 ("element"), w488) -> (w486:sgl[])
    n241 = Build Array(w525, w511, w510, w509, w508) -> (→"Encoder":sgl[])
    n242 = Build Array(w507, w506, w505, w504, w503) -> (→"DI":bool[][])
    n243 = Build Array(w499, w500, w501, w498, w497) -> (→"DO":bool[][])
    n244 = Build Array (concatenate)(w486, w472) -> (w482:sgl[])
    n245 = Array Size(array=w482) -> (size(s)=w483:i32)
    n246 = Initialize Array(sgl 0.0 ("element"), w483) -> (w485:sgl[])
    n247 = Build Array (concatenate)(w485, w471) -> (w479:sgl[])
    n248 = Array Size(array=w479) -> (size(s)=w478:i32)
    n249 = Initialize Array(sgl 0.0 ("element"), w478) -> (w480:sgl[])
    n250 = Build Array (concatenate)(w480, w470) -> (w468:sgl[])
    n251 = Array Size(array=w468) -> (size(s)=w477:i32)
    n252 = Initialize Array(sgl 0.0 ("element"), w477) -> (w476:sgl[])
    n253 = Build Array (concatenate)(w476, w469) -> (w474:sgl[])
    n254 = Build Array(w473, w472, w471, w470, w469) -> (w467:sgl[][])
    n255 = Number To Fractional String(number=w467) -> (F-format string=→"TDX ALL":string[][])  [unwired: 3 in]
    n256 = Build Array(w473, w482, w479, w468, w474) -> (→"TDX":sgl[][])
  }
  n257 = while {
    tunnel: w13 -> [w551]
    tunnel: w126 -> [w564]
    shift-right: [w556] -> _
    shift-left: w18 -> [w558]
    shift-right: [w554] -> _
    shift-left: w21 -> [w555]
    tunnel: w36 -> [w560]
    tunnel: [w561] -> w71
    shift-right: [w552] -> _
    shift-left: w21 -> [w553]
    stop <- w563 stop-if-true
    # "Logging Loop"
    n258 = call "Dequeue Message.vi"("error in (no error)"=w560, "Message Queue"=w564) -> ("error out"=w562:errorcluster, "Message Data"=w557:variant, "Message"=w565:string, "dup Message Queue"=w559:refnum<queue>)  [unwired: 6 in]
    n259 = case shown="\"Update HAL Config\"" w565 {
      tunnel: w559 -> [_ _ _ _ _ _]
      tunnel: [_ _ _ _ _ TRUE] -> w563
      tunnel: w562 -> [w569 w574 w585 w595 w601 w605]
      tunnel: [w569 w573 w584 w594 w601 w605] -> w561
      tunnel: w558 -> [w568 w571 w586 w596 w600 w604]
      tunnel: [w568 w570 w586 w596 w600 w604] -> w556
      tunnel: w557 -> [_ w572 w583 w593 _ _]
      tunnel: w555 -> [w566 w576 w580 w587 w599 w602]
      tunnel: [w566 w576 w578 w587 w599 w602] -> w554
      tunnel: w553 -> [w567 w575 w577 w589 w598 w603]
      tunnel: [w567 w575 w577 w588 w598 w603] -> w552
      tunnel: w551 -> [_ _ _ _ w597 _]
      frame Default {
      }
      frame "Update HAL Config" {
        n260 = Variant To Data(error in=w574, type=w571, Variant=w572) -> (data=w570:T1[], error out=w573:errorcluster)
      }
      frame "Start Time" {
        n261 = Variant To Data(error in=w585, type=u32 0, Variant=w583) -> (data=w581:u32, error out=w584:errorcluster)
        n262 = Get Date/Time In Seconds() -> (seconds since 1Jan1904=w579:timestamp)
        n263 = Replace Array Subset(array=w580, new element=w579, index=w581) -> (w578:timestamp[])
      }
      frame "Stop Time" {
        n264 = Variant To Data(error in=w595, type=u32 0, Variant=w593) -> (data=w591:u32, error out=w594:errorcluster)
        n265 = Get Date/Time In Seconds() -> (seconds since 1Jan1904=w590:timestamp)
        n266 = Replace Array Subset(array=w589, new element=w590, index=w591) -> (w588:timestamp[])
      }
      frame "Open Log File" {
        n267 = call "CreateLogFile.vi"("Stop Time"=w598, "Start Time"=w599, "HAL Config"=w600, "ACQ Queues"=w597) -> ()  [unwired: 8 in]
      }
      frame "EXIT" {
      }
    }
  }
  n268 = Unbundle By Name(w2) -> ("Notifiers.Acquisition.ACQ HWSync1"=w121:refnum<notifier>, "Notifiers.Control.CTRL HWSync1"=w120:refnum<notifier>, "Queues.ACQ HWSync1"=w119:refnum<queue>)
  n269 = Unbundle By Name(w2) -> ("Notifiers.Acquisition.ACQ HWSync2"=w108:refnum<notifier>, "Notifiers.Control.CTRL HWSync2"=w109:refnum<notifier>, "Queues.ACQ HWSync2"=w110:refnum<queue>)
  n270 = Unbundle By Name(w2) -> ("Notifiers.Acquisition.ACQ HWSync3"=w96:refnum<notifier>, "Notifiers.Control.CTRL HWSync3"=w97:refnum<notifier>, "Queues.ACQ HWSync3"=w98:refnum<queue>)
  n271 = Unbundle By Name(w2) -> ("Notifiers.Acquisition.ACQ HWSync4"=w101:refnum<notifier>, "Notifiers.Control.CTRL HWSync4"=w100:refnum<notifier>, "Queues.ACQ HWSync4"=w99:refnum<queue>)
  n272 = Unbundle By Name(w2) -> ("Notifiers.Acquisition.ACQ HWSync5"=w90:refnum<notifier>, "Notifiers.Control.CTRL HWSync5"=w91:refnum<notifier>, "Queues.ACQ HWSync5"=w92:refnum<queue>)
  n273 = Unbundle By Name(w24) -> ("HAL"=w49:refnum<queue>, "HWAsync10"=w50:refnum<queue>)
  n274 = Unbundle By Name(w24) -> ("HAL"=w66:refnum<queue>, "HWAsync1"=w65:refnum<queue>)
  n275 = Unbundle By Name(w24) -> ("HAL"=w61:refnum<queue>, "HWAsync2"=w62:refnum<queue>)
  n276 = Unbundle By Name(w24) -> ("HAL"=w60:refnum<queue>, "HWAsync3"=w59:refnum<queue>)
  n277 = Unbundle By Name(w24) -> ("HAL"=w55:refnum<queue>, "HWAsync4"=w56:refnum<queue>)
  n278 = Unbundle By Name(w24) -> ("HAL"=w54:refnum<queue>, "HWAsync5"=w53:refnum<queue>)
  n279 = Unbundle By Name(w24) -> ("HAL"=w37:refnum<queue>, "HWAsync6"=w38:refnum<queue>)
  n280 = Unbundle By Name(w24) -> ("HAL"=w42:refnum<queue>, "HWAsync7"=w41:refnum<queue>)
  n281 = Unbundle By Name(w24) -> ("HAL"=w43:refnum<queue>, "HWAsync8"=w44:refnum<queue>)
  n282 = Unbundle By Name(w24) -> ("HAL"=w48:refnum<queue>, "HWAsync9"=w47:refnum<queue>)
  n283 = Unbundle By Name(w24) -> ("HAL"=w131:refnum<queue>, "HWSync1"=w130:refnum<queue>)
  n284 = Unbundle By Name(w24) -> ("HAL"=w105:refnum<queue>, "HWSync2"=w106:refnum<queue>)
  n285 = Unbundle By Name(w24) -> ("HAL"=w93:refnum<queue>, "HWSync3"=w94:refnum<queue>)
  n286 = Unbundle By Name(w24) -> ("HAL"=w104:refnum<queue>, "HWSync4"=w103:refnum<queue>)
  n287 = Unbundle By Name(w24) -> ("HAL"=w87:refnum<queue>, "HWSync5"=w88:refnum<queue>)
  n288 = call "HWSyncLoop.vi"("HAL"=w131, "Index"=u32 1 ("Num of Loop"), "HWSync"=w130, "error in"=w36, "ACQ Data Queue"=w119, "CTRL Data Notifier"=w120, "ACQ Data Notifier"=w121) -> ("error out"=w86:errorcluster)  [unwired: 4 in]
  n289 = call "HWSyncLoop.vi"("HAL"=w105, "Index"=u32 2 ("Num of Loop"), "HWSync"=w106, "error in"=w36, "ACQ Data Queue"=w110, "CTRL Data Notifier"=w109, "ACQ Data Notifier"=w108) -> ("error out"=w85:errorcluster)  [unwired: 4 in]
  n290 = call "HWSyncLoop.vi"("HAL"=w93, "Index"=u32 3 ("Num of Loop"), "HWSync"=w94, "error in"=w36, "ACQ Data Queue"=w98, "CTRL Data Notifier"=w97, "ACQ Data Notifier"=w96) -> ("error out"=w84:errorcluster)  [unwired: 4 in]
  n291 = call "HWSyncLoop.vi"("HAL"=w104, "Index"=u32 4 ("Num of Loop"), "HWSync"=w103, "error in"=w36, "ACQ Data Queue"=w99, "CTRL Data Notifier"=w100, "ACQ Data Notifier"=w101) -> ("error out"=w83:errorcluster)  [unwired: 4 in]
  n292 = call "HWSyncLoop.vi"("HAL"=w87, "Index"=u32 5 ("Num of Loop"), "HWSync"=w88, "error in"=w36, "ACQ Data Queue"=w92, "CTRL Data Notifier"=w91, "ACQ Data Notifier"=w90) -> ("error out"=w82:errorcluster)  [unwired: 4 in]
  n293 = call "HWAsyncLoop.vi"("HAL"=w66, "Index"=u32 1, "HWAsync"=w65, "error in"=w36, "Async ACQ Notifier in"=w12) -> ("error out"=w35:errorcluster)  [unwired: 6 in]
  n294 = call "HWAsyncLoop.vi"("HAL"=w61, "Index"=u32 2, "HWAsync"=w62, "error in"=w36, "Async ACQ Notifier in"=w11) -> ("error out"=w33:errorcluster)  [unwired: 6 in]
  n295 = call "HWAsyncLoop.vi"("HAL"=w60, "Index"=u32 3, "HWAsync"=w59, "error in"=w36, "Async ACQ Notifier in"=w10) -> ("error out"=w32:errorcluster)  [unwired: 6 in]
  n296 = call "HWAsyncLoop.vi"("HAL"=w55, "Index"=u32 4, "HWAsync"=w56, "error in"=w36, "Async ACQ Notifier in"=w9) -> ("error out"=w31:errorcluster)  [unwired: 6 in]
  n297 = call "HWAsyncLoop.vi"("HAL"=w54, "Index"=u32 5, "HWAsync"=w53, "error in"=w36, "Async ACQ Notifier in"=w8) -> ("error out"=w30:errorcluster)  [unwired: 6 in]
  n298 = call "HWAsyncLoop.vi"("HAL"=w37, "Index"=u32 6, "HWAsync"=w38, "error in"=w36, "Async ACQ Notifier in"=w7) -> ("error out"=w29:errorcluster)  [unwired: 6 in]
  n299 = call "HWAsyncLoop.vi"("HAL"=w42, "Index"=u32 7, "HWAsync"=w41, "error in"=w36, "Async ACQ Notifier in"=w6) -> ("error out"=w28:errorcluster)  [unwired: 6 in]
  n300 = call "HWAsyncLoop.vi"("HAL"=w43, "Index"=u32 8, "HWAsync"=w44, "error in"=w36, "Async ACQ Notifier in"=w5) -> ("error out"=w27:errorcluster)  [unwired: 6 in]
  n301 = call "HWAsyncLoop.vi"("HAL"=w48, "Index"=u32 9, "HWAsync"=w47, "error in"=w36, "Async ACQ Notifier in"=w4) -> ("error out"=w26:errorcluster)  [unwired: 6 in]
  n302 = call "HWAsyncLoop.vi"("HAL"=w49, "Index"=u32 10, "HWAsync"=w50, "error in"=w36, "Async ACQ Notifier in"=w3) -> ("error out"=w25:errorcluster)  [unwired: 6 in]
  n303 = Merge Errors(w35, w33, w32, w31, w30, w29, w28, w27, w26, w25) -> (w34:errorcluster)
  n304 = Set Occurrence(w112) -> ()
  n305 = Merge Errors(w86, w85, w84, w83, w82, w34) -> (w70:errorcluster)
  n306 = Merge Errors(w129, w69, w70, w71) -> (w117:errorcluster)
  n307 = call "Destroy All Data Queues.vi"("Error In"=w117, "WINFAS 2 Data Queue.lvlib:All Data Queues Cluster"=w2) -> ("Error Out"=w116:errorcluster)  [unwired: 9 in]
  n308 = call "Destroy All Message Queues.vi"("error in (no error)"=w116, "Message Queues Out"=w24) -> ("error out"=w115:errorcluster)  [unwired: 9 in]
  n309 = property class="App"(error in=w115) -> ("App.Kind"=w125:T2)  [unwired: 1 in, 2 out]
  n310 = case shown="\"Development System\"" w125 {
    tunnel: [TRUE FALSE TRUE] -> w124
    tunnel: [w607 w621 w627] -> _
    frame "invalid app kind", Default {
      n311 = property class="VI"() -> (error out=w608:errorcluster, "Panel"=w618:refnum<vi>)  [unwired: 2 in, 1 out]
      n312 = property class="Pnl"(reference=w618, error in=w608) -> (error out=w609:errorcluster, "AllObjs[]"=w617:refnum<vi>[])  [unwired: 1 out]
      n313 = control-ref of="This VI"() -> (w615:refnum<vi>)
      n314 = Close Reference(reference=w617, error in (no error)=w609) -> (error out=w614:errorcluster)
      n315 = invoke class="VI" method="FP.Close"(reference=w615, error in=w614) -> (reference out=w613:refnum<vi>, error out=w612:errorcluster)  [unwired: 1 in, 1 out]
      n316 = invoke class="VI" method="Abort VI"(reference=w613, error in=w612) -> (reference out=w610:refnum<vi>, error out=w611:errorcluster)  [unwired: 1 in, 1 out]
      n317 = Close Reference(reference=w610, error in (no error)=w611) -> (error out=w619:errorcluster)
      n318 = control-ref of="This Application"() -> (w620:refnum<vi>)
      n319 = Close Reference(reference=w620, error in (no error)=w619) -> (error out=w607:errorcluster)
    }
    frame "Development System" {
      n320 = property class="VI"() -> (error out=w622:errorcluster, "Panel"=w626:refnum<vi>)  [unwired: 2 in, 1 out]
      n321 = property class="Pnl"(reference=w626, error in=w622) -> (error out=w623:errorcluster, "AllObjs[]"=w625:refnum<vi>[])  [unwired: 1 out]
      n322 = Close Reference(reference=w625, error in (no error)=w623) -> (error out=w621:errorcluster)
    }
    frame "Run Time System" {
      n323 = property class="VI"() -> (error out=w628:errorcluster, "Panel"=w638:refnum<vi>)  [unwired: 2 in, 1 out]
      n324 = property class="Pnl"(reference=w638, error in=w628) -> (error out=w629:errorcluster, "AllObjs[]"=w637:refnum<vi>[])  [unwired: 1 out]
      n325 = control-ref of="This VI"() -> (w635:refnum<vi>)
      n326 = Close Reference(reference=w637, error in (no error)=w629) -> (error out=w634:errorcluster)
      n327 = invoke class="VI" method="FP.Close"(reference=w635, error in=w634) -> (reference out=w633:refnum<vi>, error out=w632:errorcluster)  [unwired: 1 in, 1 out]
      n328 = invoke class="VI" method="Abort VI"(reference=w633, error in=w632) -> (reference out=w630:refnum<vi>, error out=w631:errorcluster)  [unwired: 1 in, 1 out]
      n329 = Close Reference(reference=w630, error in (no error)=w631) -> (error out=w639:errorcluster)
      n330 = control-ref of="This Application"() -> (w640:refnum<vi>)
      n331 = Close Reference(reference=w640, error in (no error)=w639) -> (error out=w627:errorcluster)
    }
  }
  n332 = Quit LabVIEW(quit? (T)=w124) -> ()
